vi "channel_model.vi"(8 "error in (no error)":errorcluster, 10 "Channel Model Parameters":T1) -> (0 "error out":errorcluster)   [LabVIEW 2012]
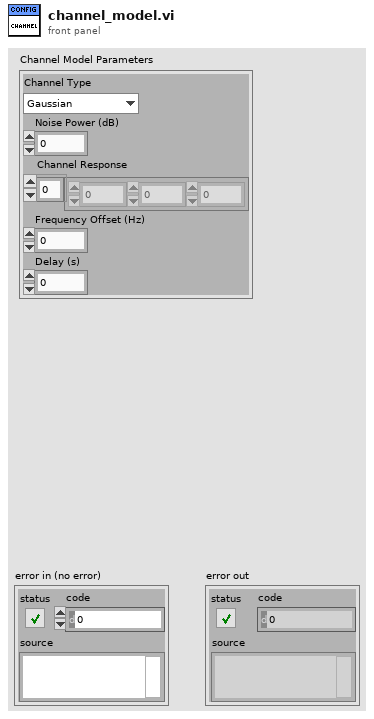
[diagram p1: front panel]
types:
  T1 = cluster{"Channel Type":enum16{"Gaussian", "ISI"}, "Noise Power (dB)":dbl, "Channel Response":cdb[], "Frequency Offset (Hz)":dbl, "Delay (s)":dbl}
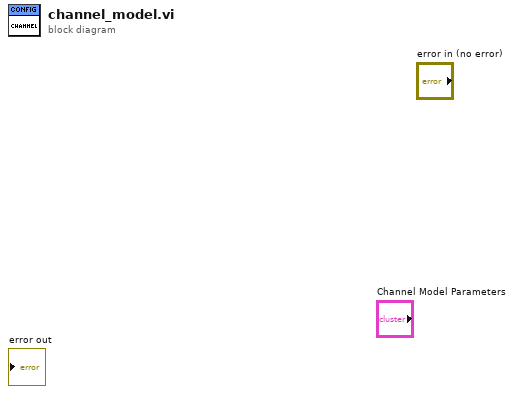
[diagram p0: block diagram]
diagram:
